vi "Set document.vi"(8 "error in (no error)":errorcluster caption="entrée d'erreur (pas d'erreur)", 11 "Firebase (Default) en entrée":refnum<class "Firebase Driver.lvclass">) -> (0 "error out":errorcluster caption="sortie d'erreur", 3 "Firebase (Default) en sortie":refnum<class "Firebase Driver.lvclass">)   [LabVIEW 2020, in "Library Instrument & Equipement.lvlib" / "Library FireBase.lvlib" / "Firebase Driver.lvclass"]
uses:
  Firebase Driver.lvclass
  Commun VI/TypeDef/Liste Error.ctl
  Firebase Driver.lvclass/Firebase Driver.ctl
  JSON API/JSON Value/Set from JSON string.vi
  JSON API/JSON Object/JSON Object.lvclass
  C:/Users/ngarcin/OneDrive - Altyor/Standard TB/Class/JSON API/JSON Value/JSON Value.lvclass
  JSON API/Variant JSON/Add Variant to JSON Object.vi
  JSON API/JSON Value/Get Item by name array.vi
  <vilib>/httpClient/POSTBuffer.vi
  JSON API/JSON Value/JSON Value.lvclass
  JSON API/Get Polymorphic/JSON GetSet.lvlib
  <vilib>/httpClient/LabVIEWHTTPClient.lvlib
  JSON API/Variant JSON/Variant JSON.lvlib
  Commun VI/Library Commun.lvlib
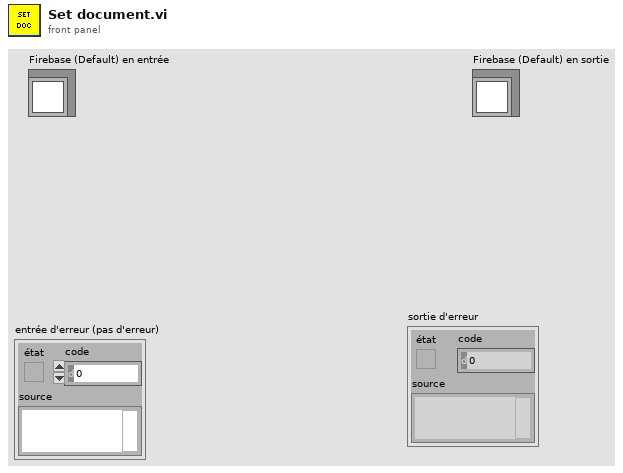
[diagram p1: front panel]
types:
  T1 = typedef "Library Commun.lvlib/Liste Error.ctl" = enum16{"Firebase Driver - Get Document", "Firebase Driver - Get Document With Where", "Firebase Driver - Delete Document", "Firebase Driver - Set Document", "Firebase Driver - Update Document", "Firebase Altyor - Search Document Bench", "Firebase Altyor - Class Not in Firebase", "Spectrum_Analyser - Timeout", "Relay Board - Qty Relay", "DIO - Pb Funtion", "Power_Supply - Peripherical not find", "Mutimeter - Peripherical not find", "Instrument - Function Not Used", "Instrument - Instrument name not specified", "Instrument - Allready Initialised", "Instrument - TimeOut", "Instrument - the instrument must be Initialise before", "Instrument - Frame Not received", "Instrument - Frame Nok", "Test - Initialise the File_for_Save", "Test - Timeout", "Test - Cmd Error", "FGV - Variable ", "BDD FireBase - Define Class", "SN - Class Not Define"}
  T2 = typedef "LabVIEWHTTPClient.lvlib/ClientHandle.ctl" = refnum<k1>
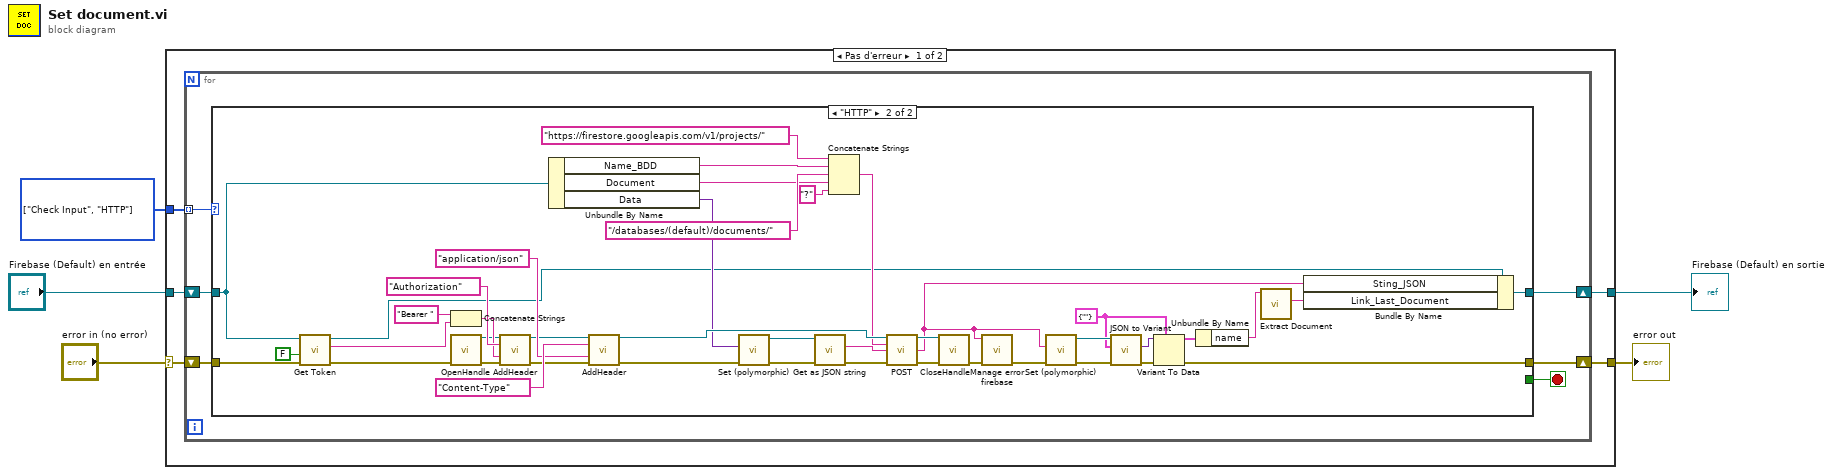
[diagram p0: block diagram]
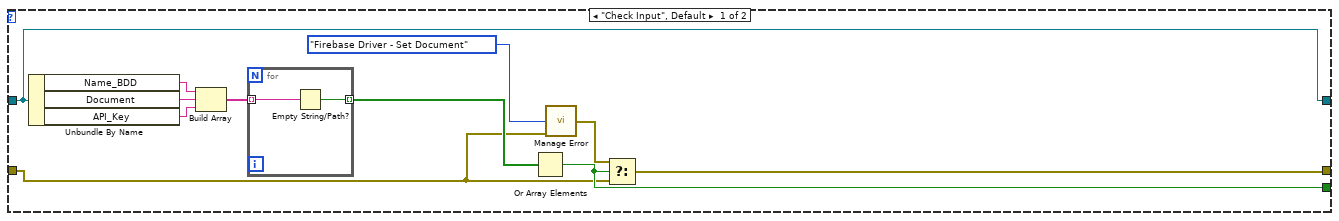
[diagram p2: hidden frame]
diagram:
  w1 = enum16{"Check Input", "HTTP"}[] [enum."Check Input", enum."HTTP"] items=["Check Input", "HTTP"]
  n1 = case shown="Pas d'erreur" "error in (no error)" {
    selector: "error in (no error)" -> [w10 w74]
    tunnel: [w9 w74] -> w4
    tunnel: "Firebase (Default) en entrée" -> [w8 w73]
    tunnel: [w7 w73] -> w2
    tunnel: w1 -> [w6 _]
    frame No Error {
      n2 = for {
        shift-right: [w13] -> w9
        shift-left: w10 -> [w16]
        shift-right: [w14] -> w7
        shift-left: w8 -> [w15]
        tunnel: w6 -> [w12] mode=indexing
        stop <- w11 stop-if-true
        n3 = case shown="\"HTTP\"" w12 {
          tunnel: w16 -> [w17 w57]
          tunnel: w15 -> [w23 w35]
          tunnel: [w23 w51] -> w14
          tunnel: [w24 w42] -> w13
          tunnel: [w25 _] -> w11
          frame "Check Input", Default {
            n4 = Unbundle By Name(w23) -> ("Name_BDD"=w22:string, "Document"=w21:string, "API_Key"=w20:string)
            n5 = Build Array(w22, w21, w20) -> (w27:string[])
            n6 = for {
              tunnel: w27 -> [w28] mode=indexing
              tunnel: [w29] -> w26 mode=indexing
              n7 = Empty String/Path?(string/path=w28) -> (empty?=w29:bool)
            }
            n8 = Or Array Elements(Boolean array=w26) -> (logical OR=w25:bool)
            n9 = call "Manage Error.vi"("Code Erreur"=Liste_Error."Firebase Driver - Set Document", "error in (no error)"=w17) -> ("error out"=w18:errorcluster)  [unwired: 13 in]
            n10 = Select(t=w18, s=w25, f=w17) -> (s? t:f=w24:errorcluster)
          }
          frame "HTTP" {
            w46 = cluster{"name":string} {"name"=""}
            n11 = call-dynamic "Get Token.vi"("error in (no error)"=w57, "Reset"=FALSE, "Build Library FireBase.lvlib:Firebase (Default) IN"=w35) -> ("error out"=w56:errorcluster, "idToken"=w36:string, "Build Library FireBase.lvlib:Firebase (Default) Out"=w34:refnum<class "Firebase Driver.lvclass">)  [unwired: 6 in]
            n12 = Concatenate Strings("Bearer " ("chaîne"), w36) -> (w63:string)
            n13 = call <vilib>:"OpenHandle.vi"("error in (no error)"=w56) -> ("client handle out"=w61:T2, "error out"=w62:errorcluster)  [unwired: 13 in]
            n14 = call <vilib>:"AddHeader.vi"("client handle"=w61, "header"="Authorization", "value"=w63, "error in (no error)"=w62) -> ("client handle out"=w66:T2, "error out"=w67:errorcluster)  [unwired: 10 in]
            n15 = Unbundle By Name(w35) -> ("Name_BDD"=w58:string, "Document"=w33:string, "Data"=w52:variant)
            n16 = call <vilib>:"AddHeader.vi"("client handle"=w66, "header"="Content-Type", "value"="application/json", "error in (no error)"=w67) -> ("client handle out"=w59:T2, "error out"=w55:errorcluster)  [unwired: 10 in]
            n17 = call-poly "Set (polymorphic).vi"("error in (no error)"=w55, "Variant"=w52) -> ("error out"=w39:errorcluster, "JSON Object out"=w40:refnum<class "JSON Object.lvclass">)  [unwired: 8 in]
            n18 = call "Get as JSON string.vi"("error in (no error)"=w39, "JSON Value in"=w40) -> ("error out"=w38:errorcluster, "<JSON>"=w37:string)  [unwired: 8 in]
            n19 = Concatenate Strings("https://firestore.googleapis.com/v1/projects/" ("string"), w58, "/databases/(default)/documents/" ("string"), w33, "?" ("chaîne")) -> (w41:string)
            n20 = call-poly <vilib>:"POST.vi"("client handle"=w59, "url"=w41, "buffer"=w37, "error in (no error)"=w38) -> ("client handle out"=w70:T2, "body"=w31:string, "error out"=w71:errorcluster)  [unwired: 8 in, 1 out]
            n21 = call <vilib>:"CloseHandle.vi"("client handle"=w70, "error in (no error)"=w71) -> ("error out"=w60:errorcluster)  [unwired: 13 in]
            n22 = call "Manage error firebase.vi"("error in (no error)"=w60, "Body"=w31) -> ("error out"=w43:errorcluster)  [unwired: 9 in]
            n23 = call-poly "Set (polymorphic).vi"("error in (no error)"=w43, "JSON stream"=w31) -> ("error out"=w47:errorcluster, "JSON Value out"=w50:refnum<class "JSON Value.lvclass">)  [unwired: 7 in, 1 out]
            n24 = call "JSON to Variant.vi"("error in (no error)"=w47, "Variant (Data Type)"=w46, "JSON Value"=w50) -> ("error out"=w48:errorcluster, "Variant out"=w49:variant)  [unwired: 7 in]
            n25 = Variant To Data(error in=w48, type=w46, Variant=w49) -> (data=w45:cluster{"name":string}, error out=w42:errorcluster)
            n26 = Unbundle By Name(w45) -> ("name"=w44:string)
            n27 = call "Extract Document.vi"("Name"=w44) -> ("Source"=w32:string)  [unwired: 9 in, 1 out]
            n28 = Bundle By Name(cluster=w34, "Sting_JSON"=w31, "Link_Last_Document"=w32) -> (w51:refnum<class "Firebase Driver.lvclass">)
          }
        }
      }
    }
    frame Error {
    }
  }
  "error out" <- w4
  "Firebase (Default) en sortie" <- w2
